vi "comet_thermo_get_idn_HTTP.vi"(8 "error in":errorcluster, 10 "timeout (5000)":i32=5000, 11 "IP":string) -> (0 "error out":errorcluster, 1 "name":string, 2 "serial":string, 3 "type":string, 4 "fw rev.":string, 5 "ID string (virtual)":string, 6 "www rev.":string)   [LabVIEW 2020]
uses:
  <vilib>/httpClient/LabVIEWHTTPClient.lvlib
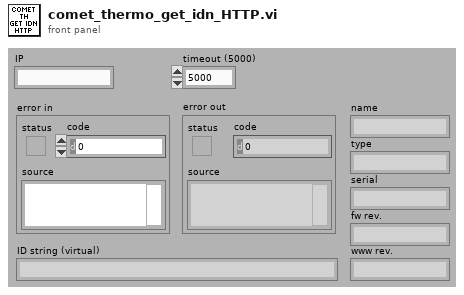
[diagram p1: front panel]
types:
  T1 = typedef "LabVIEWHTTPClient.lvlib/ClientHandle.ctl" = refnum<k1>
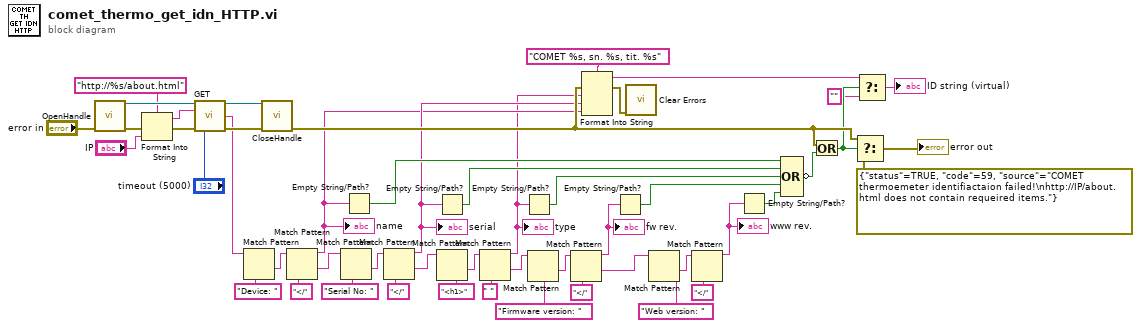
[diagram p0: block diagram]
diagram:
  n1 = call <vilib>:"OpenHandle.vi"("error in (no error)"="error in") -> ("client handle out"=w50:T1, "error out"=w47:errorcluster)  [unwired: 13 in]
  n2 = Format Into String(format string="http://%s/about.html", error in=w47, "IP") -> (resulting string=w45:string, error out=w48:errorcluster)  [unwired: 1 in]
  n3 = call <vilib>:"GET.vi"("client handle"=w50, "url"=w45, "error in (no error)"=w48, "timeout (10000)"="timeout (5000)") -> ("client handle out"=w42:T1, "body"=w41:string, "error out"=w43:errorcluster)  [unwired: 8 in, 1 out]
  n4 = Match Pattern(string=w41, regular expression="Device: ") -> (after substring=w39:string)  [unwired: 1 in, 3 out]
  n5 = call <vilib>:"CloseHandle.vi"("client handle"=w42, "error in (no error)"=w43) -> ("error out"=w9:errorcluster)  [unwired: 13 in]
  n6 = Match Pattern(string=w39, regular expression="</") -> (before substring=w6:string, after substring=w33:string)  [unwired: 1 in, 2 out]
  "name" <- w6
  n7 = Match Pattern(string=w33, regular expression="Serial No: ") -> (after substring=w35:string)  [unwired: 1 in, 3 out]
  n8 = Empty String/Path?(string/path=w6) -> (empty?=w20:bool)
  n9 = Match Pattern(string=w35, regular expression="</") -> (before substring=w7:string, after substring=w30:string)  [unwired: 1 in, 2 out]
  "serial" <- w7
  n10 = Empty String/Path?(string/path=w7) -> (empty?=w21:bool)
  n11 = Match Pattern(string=w30, regular expression="<h1>") -> (after substring=w31:string)  [unwired: 1 in, 3 out]
  n12 = Match Pattern(string=w31, regular expression=" ") -> (before substring=w5:string, after substring=w24:string)  [unwired: 1 in, 2 out]
  "type" <- w5
  n13 = Empty String/Path?(string/path=w5) -> (empty?=w22:bool)
  n14 = Match Pattern(string=w24, regular expression="Firmware version: ") -> (after substring=w26:string)  [unwired: 1 in, 3 out]
  n15 = Match Pattern(string=w26, regular expression="</") -> (before substring=w28:string, after substring=w16:string)  [unwired: 1 in, 2 out]
  "fw rev." <- w28
  n16 = Format Into String(format string="COMET %s, sn. %s, tit. %s", error in=w9, w5, w7, w6) -> (resulting string=w2:string, error out=w8:errorcluster)  [unwired: 1 in]
  n17 = Empty String/Path?(string/path=w28) -> (empty?=w23:bool)
  n18 = call <vilib>:"Clear Errors.vi"("error in (no error)"=w8) -> ()  [unwired: 5 in, 2 out]
  n19 = Match Pattern(string=w16, regular expression="Web version: ") -> (after substring=w18:string)  [unwired: 1 in, 3 out]
  n20 = Match Pattern(string=w18, regular expression="</") -> (before substring=w15:string)  [unwired: 1 in, 3 out]
  "www rev." <- w15
  n21 = Empty String/Path?(string/path=w15) -> (empty?=w14:bool)
  n22 = Compound Arithmetic op=OR(w20, w21, w22, w23, w14) -> (invert w13:bool)
  n23 = Or(x=w9, y=w13) -> (x .or. y?=w3:bool)
  n24 = Select(t=w9, s=w3, f=errorcluster {"status"=TRUE, "code"=59, "source"="COMET thermoemeter identifiactaion failed!\nhttp://IP/about.html does not contain requeired items."}) -> (s? t:f=→"error out":errorcluster)
  n25 = Select(t=w2, s=w3, f="") -> (s? t:f=→"ID string (virtual)":string)
